vi "Data Group RW.vi"(6 "section":string="info", 7 "Operate":enum16{"Read", "Write"}(ring), 8 "Error In":errorcluster, 10 "Source Path":path caption="配置文件的路径", 11 "Group Type In":T1) -> (0 "Error Out":errorcluster, 1 "Data":string[](array[string]), 2 "Name":string[](array[string]), 3 "Group Type Out":T1)   [LabVIEW 2020]
uses:
  0007 Controls/002 Group Type.ctl
  b1f5c254-8b2e-415b-9e48-2b3ded4d4a7a.vi
  <vilib>/Utility/config.llb/Open Config Data.vi
  <vilib>/Utility/config.llb/Read Key.vi
  <vilib>/Utility/config.llb/Read Key (String).vi
  <vilib>/Utility/config.llb/Write Key.vi
  <vilib>/Utility/config.llb/Write Key (String).vi
  <vilib>/Utility/config.llb/Close Config Data.vi
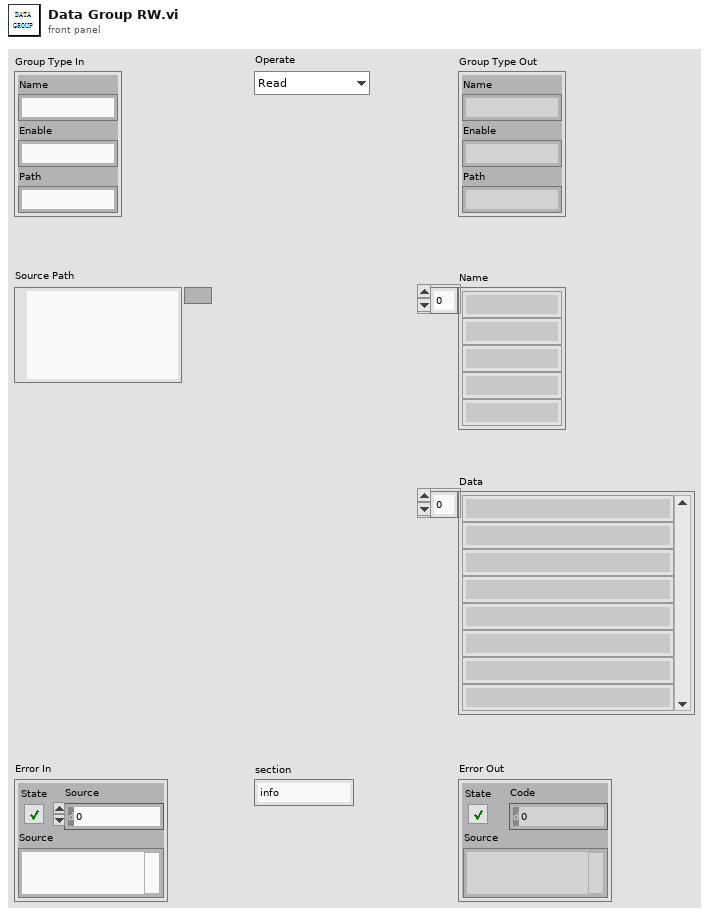
[diagram p1: front panel]
types:
  T1 = typedef "002 Group Type.ctl" = cluster{"Name":string, "Enable":string, "Path":string}
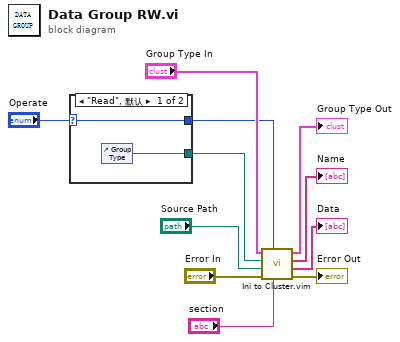
[diagram p0: block diagram]
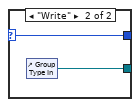
[diagram p2: hidden frame]
diagram:
  n1 = case shown="\"Read\", 默认" "Operate" {
    selector: "Operate" -> [w12 w15]
    tunnel: [w13 w14] -> w1
    tunnel: [w12 w15] -> w2
    frame "Read", Default {
      n2 = control-ref of="Group Type"() -> (w13:refnum<vi>)
    }
    frame "Write" {
      n3 = control-ref of="Group Type In"() -> (w14:refnum<vi>)
    }
  }
  n4 = call "Ini to Cluster.vim"("section"="section", "Operate"=w2, "Error In"="Error In", "Source Path"="Source Path", "Cluster Ref In"=w1, "Cluster Type In"="Group Type In") -> ("Error Out"=→"Error Out":errorcluster, "Data"=→"Data":string[], "Name"=→"Name":string[], "Cluster Out"=→"Group Type Out":T1)  [unwired: 2 in]
